vi "Signals (Read).vi"   [LabVIEW 2013, in "Mercury iXX.lvlib"]
doc: "Read the signal data of any devices within the Mercury Instrument."
uses:
  <instrlib>/Mercury iXX/Mercury iXX.lvlib
  <instrlib>/Mercury iXX/Public/Libraries/Temperature.lvlib
  <instrlib>/Mercury iXX/Public/Libraries/Heater.lvlib
  <instrlib>/Mercury iXX/Public/Libraries/Level Meter.lvlib
  <instrlib>/Mercury iXX/Public/Libraries/Auxiliary.lvlib
  <instrlib>/Mercury iXX/Public/Libraries/Magnet.lvlib
  <instrlib>/Mercury iXX/Public/Libraries/Flow.lvlib
  <instrlib>/Mercury iXX/Public/Libraries/Pressure.lvlib
  <instrlib>/Mercury iXX/Public/Libraries/Lambda.lvlib
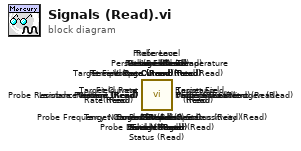
[diagram p0: block diagram]
diagram:
  n1 = call <instrlib>:"Lambda Valve Open Percent (Read).vi"() -> ()  [unwired: 7 in, 5 out]
  n2 = call <instrlib>:"Lambda Temperature (Read).vi"() -> ()  [unwired: 7 in, 5 out]
  n3 = call <instrlib>:"Lambda Pressure (Read).vi"() -> ()  [unwired: 7 in, 5 out]
  n4 = call <instrlib>:"PSU Status (Read).vi"() -> ()  [unwired: 6 in, 6 out]
  n5 = call <instrlib>:"Voltage (Read).vi"() -> ()  [unwired: 7 in, 5 out]
  n6 = call <instrlib>:"Pressure (Read).vi"() -> ()  [unwired: 7 in, 5 out]
  n7 = call <instrlib>:"Power (Read).vi"() -> ()  [unwired: 7 in, 5 out]
  n8 = call <instrlib>:"Current (Read).vi"() -> ()  [unwired: 7 in, 5 out]
  n9 = call <instrlib>:"Voltage (Read).vi"() -> ()  [unwired: 7 in, 5 out]
  n10 = call <instrlib>:"Power (Read).vi"() -> ()  [unwired: 7 in, 5 out]
  n11 = call <instrlib>:"Current (Read).vi"() -> ()  [unwired: 7 in, 5 out]
  n12 = call <instrlib>:"Reference (Read).vi"() -> ()  [unwired: 7 in, 5 out]
  n13 = call <instrlib>:"PSU Action Status (Read).vi"() -> ()  [unwired: 8 in, 4 out]
  n14 = call <instrlib>:"Switch Heater Status (Read).vi"() -> ()  [unwired: 8 in, 4 out]
  n15 = call <instrlib>:"Target Field Rate (Read).vi"() -> ()  [unwired: 7 in, 5 out]
  n16 = call <instrlib>:"Target Current Rate (Read).vi"() -> ()  [unwired: 7 in, 5 out]
  n17 = call <instrlib>:"Target Field (Read).vi"() -> ()  [unwired: 7 in, 5 out]
  n18 = call <instrlib>:"Target Current (Read).vi"() -> ()  [unwired: 7 in, 5 out]
  n19 = call <instrlib>:"Persistant Field (Read).vi"() -> ()  [unwired: 7 in, 5 out]
  n20 = call <instrlib>:"Persistant Current (Read).vi"() -> ()  [unwired: 7 in, 5 out]
  n21 = call <instrlib>:"Field Rate (Read).vi"() -> ()  [unwired: 7 in, 5 out]
  n22 = call <instrlib>:"Field (Read).vi"() -> ()  [unwired: 7 in, 5 out]
  n23 = call <instrlib>:"Current Rate (Read).vi"() -> ()  [unwired: 7 in, 5 out]
  n24 = call <instrlib>:"Current (Read).vi"() -> ()  [unwired: 7 in, 5 out]
  n25 = call <instrlib>:"Voltage (Read).vi"() -> ()  [unwired: 7 in, 5 out]
  n26 = call <instrlib>:"Percent Open (Read).vi"() -> ()  [unwired: 7 in, 5 out]
  n27 = call <instrlib>:"Position (Read).vi"() -> ()  [unwired: 7 in, 5 out]
  n28 = call <instrlib>:"Probe Level Nitrogen (Read).vi"() -> ()  [unwired: 7 in, 5 out]
  n29 = call <instrlib>:"Probe Frequency Nitrogen (Read).vi"() -> ()  [unwired: 7 in, 5 out]
  n30 = call <instrlib>:"Probe Count Nitrogen (Read).vi"() -> ()  [unwired: 7 in, 5 out]
  n31 = call <instrlib>:"Probe Level Helium (Read).vi"() -> ()  [unwired: 7 in, 5 out]
  n32 = call <instrlib>:"Probe Resistance Helium (Read).vi"() -> ()  [unwired: 7 in, 5 out]
  n33 = call <instrlib>:"Current (Read).vi"() -> ()  [unwired: 7 in, 5 out]
  n34 = call <instrlib>:"Power (Read).vi"() -> ()  [unwired: 7 in, 5 out]
  n35 = call <instrlib>:"Voltage (Read).vi"() -> ()  [unwired: 7 in, 5 out]
  n36 = call <instrlib>:"Temperature Sensitivity (Read).vi"() -> ()  [unwired: 7 in, 5 out]
  n37 = call <instrlib>:"Temperature (Read).vi"() -> ()  [unwired: 7 in, 5 out]
  n38 = call <instrlib>:"Resistance (Read).vi"() -> ()  [unwired: 7 in, 5 out]
  n39 = call <instrlib>:"Power (Read).vi"() -> ()  [unwired: 7 in, 5 out]
  n40 = call <instrlib>:"Current (Read).vi"() -> ()  [unwired: 7 in, 5 out]
  n41 = call <instrlib>:"Voltage (Read).vi"() -> ()  [unwired: 7 in, 5 out]
